vi "A33ConfigureAM.vi"(0 "VISA resource name":refnum<visa-resource-name>, 1 "Enable Amplitude Modulation (T:Enable)":bool=TRUE, 2 "Modulation Frequency (1000.0 Hz)":dbl=1000.0 format="%#_12g", 5 "Channel (1: Channel1)":u16(ring)=1 items=["Channel1"=1, "Channel2"=2], 7 "AM Source (0: Internal)":u16(ring) items=["Internal", "External", "Channel 1", "Channel 2"], 9 "Modulation Waveform (0: Sine)":u16(ring) items=["Sine", "Square", "Triangle", "Ramp", "Negative Ramp", "Noise", "PRBS", "ARB"], 11 "error in (no error)":errorcluster, 13 "Modulation Depth (100.0 %)":dbl=100.0 format="%#_12g", 14 "Enable Carrier Suppression (F: Disable)":bool) -> (4 "VISA resource name out":refnum<visa-resource-name>, 15 "error out":errorcluster)   [LabVIEW 2022 SP3]
doc: "Configures and enables amplitude modulation (AM). In AM, the amplitude of the carrier is varied by the amplitude of the modulating waveform. \n\n<B>Note:</B> The carrier waveform shape and parameters are set by the Configure Standard Waveform VI."
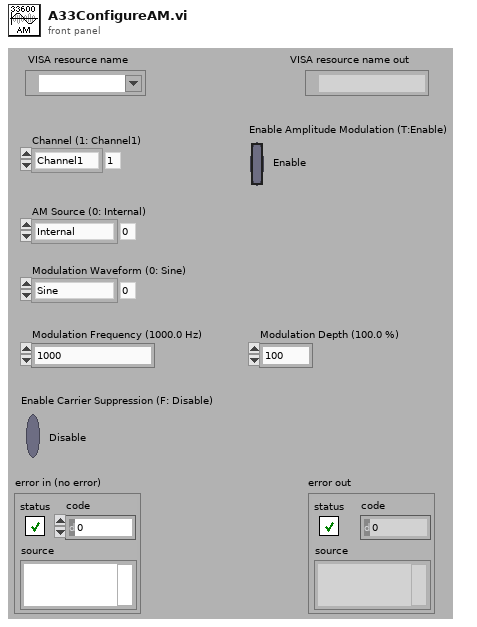
[diagram p1: front panel]
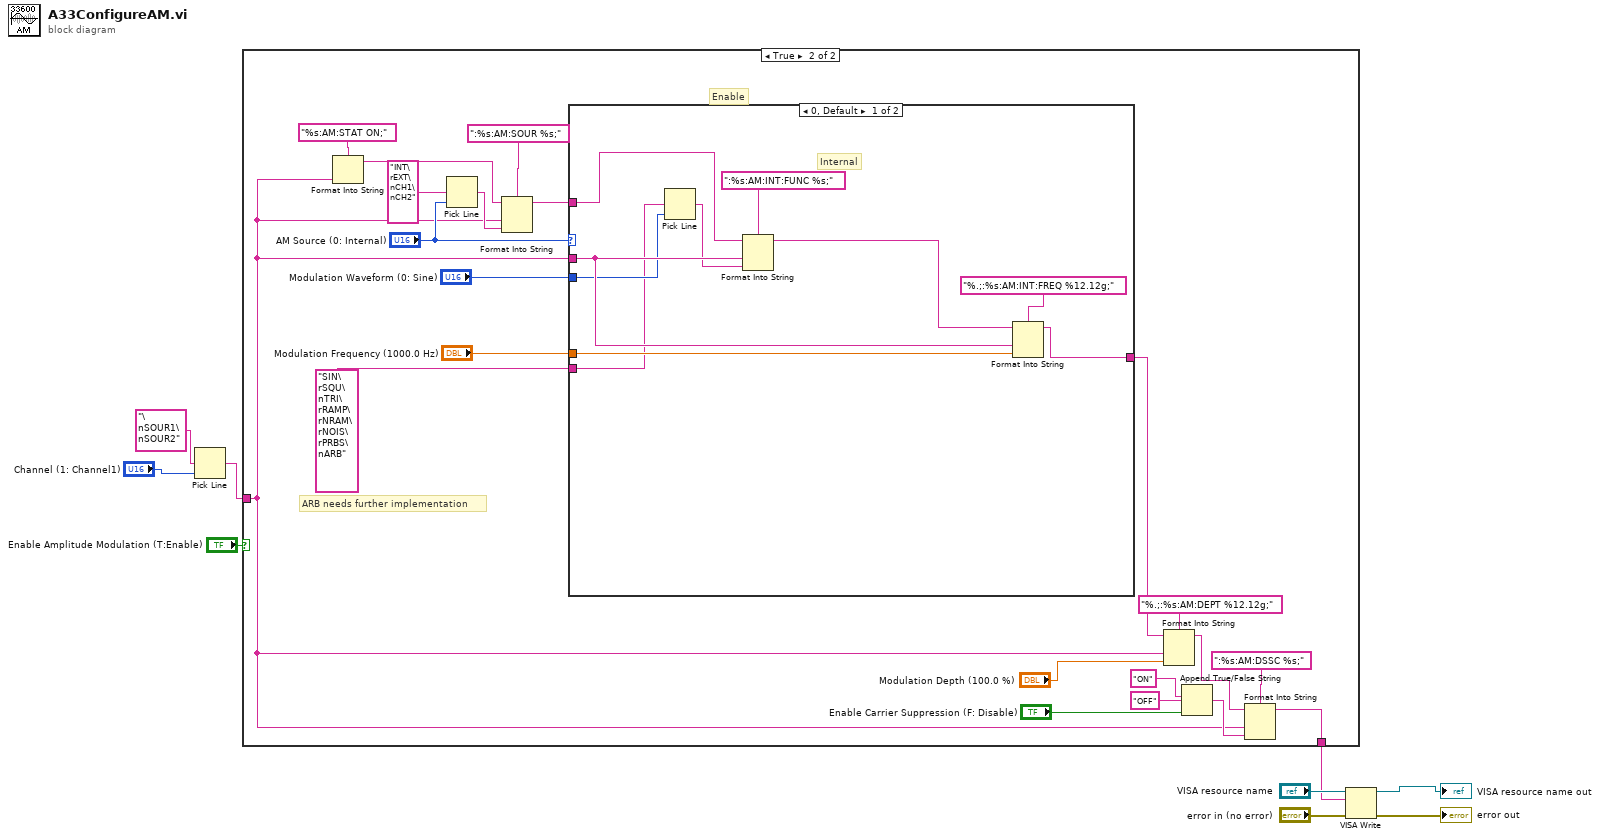
[diagram p0: block diagram]
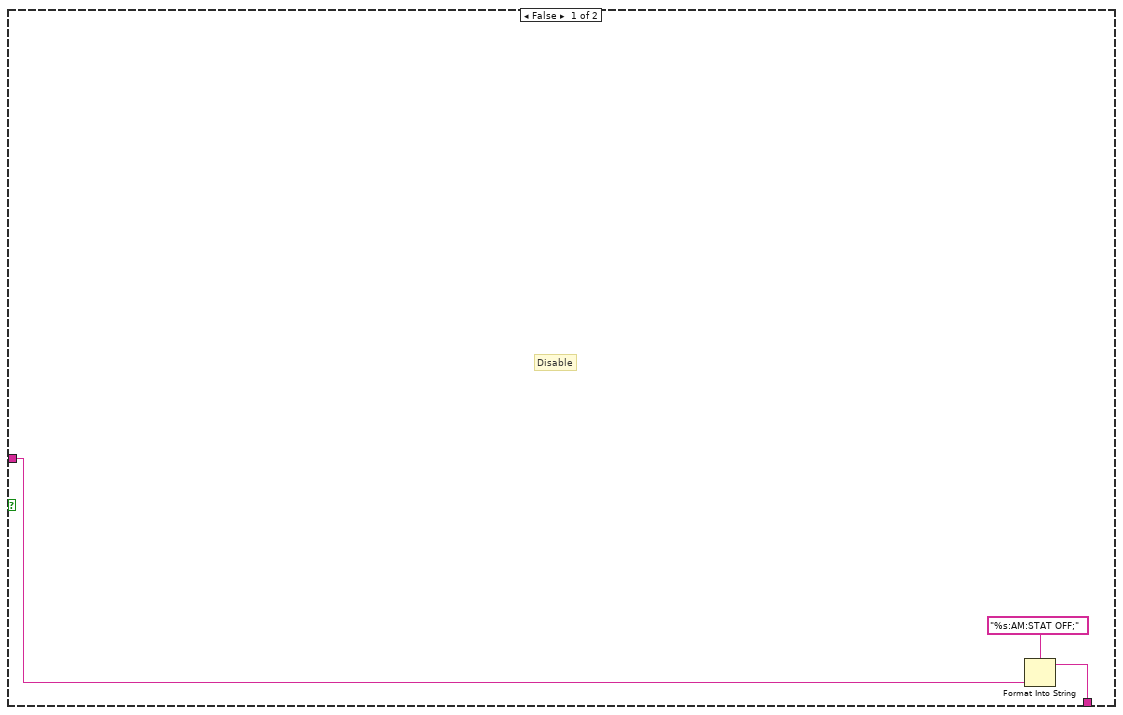
[diagram p2: hidden frame]
diagram:
  n1 = Pick Line(multi-line string="\nSOUR1\nSOUR2" ("string (\"\")"), line index="Channel (1: Channel1)") -> (output string=w1:string)  [unwired: 1 in]
  n2 = case shown="True" "Enable Amplitude Modulation (T:Enable)" {
    tunnel: [w11 w15] -> w7
    tunnel: w1 -> [w10 w13]
    frame False {
      # "Disable"
      n3 = Format Into String(format string="%s:AM:STAT OFF;", w10) -> (resulting string=w11:string)  [unwired: 2 in, 1 out]
    }
    frame True {
      # "ARB needs further implementation"
      # "Enable"
      n4 = Format Into String(format string="%s:AM:STAT ON;", w13) -> (resulting string=w16:string)  [unwired: 2 in, 1 out]
      n5 = Pick Line(multi-line string="INT\rEXT\nCH1\nCH2", line index="AM Source (0: Internal)") -> (output string=w18:string)  [unwired: 1 in]
      n6 = Format Into String(format string=":%s:AM:SOUR %s;", initial string=w16, w13, w18) -> (resulting string=w20:string)  [unwired: 1 in, 1 out]
      n7 = case shown="0, Default" "AM Source (0: Internal)" {
        tunnel: w13 -> [w39 _]
        tunnel: [w41 w44] -> w32
        tunnel: "Modulation Waveform (0: Sine)" -> [w36 _]
        tunnel: "Modulation Frequency (1000.0 Hz)" -> [w40 _]
        tunnel: w20 -> [w37 w44]
        tunnel: "SIN\rSQU\nTRI\rRAMP\rNRAM\rNOIS\rPRBS\nARB" -> [w35 _]
        frame 0, Default {
          # "Internal"
          n8 = Pick Line(multi-line string=w35, line index=w36) -> (output string=w38:string)  [unwired: 1 in]
          n9 = Format Into String(format string=":%s:AM:INT:FUNC %s;", initial string=w37, w39, w38) -> (resulting string=w34:string)  [unwired: 1 in, 1 out]
          n10 = Format Into String(format string="%.;:%s:AM:INT:FREQ %12.12g;", initial string=w34, w39, w40) -> (resulting string=w41:string)  [unwired: 1 in, 1 out]
        }
        frame 1..3 {
          # "Other Channel or External"
        }
      }
      n11 = Format Into String(format string="%.;:%s:AM:DEPT %12.12g;", initial string=w32, w13, "Modulation Depth (100.0 %)") -> (resulting string=w28:string)  [unwired: 1 in, 1 out]
      n12 = Append True/False String(1:"Enable Carrier Suppression (F: Disable)", 2:"OFF", 3:"ON") -> (0:w23:string)  [unwired: 1 in]
      n13 = Format Into String(format string=":%s:AM:DSSC %s;", initial string=w28, w13, w23) -> (resulting string=w15:string)  [unwired: 1 in, 1 out]
    }
  }
  n14 = VISA Write(VISA resource name="VISA resource name", write buffer=w7, error in (no error)="error in (no error)") -> (VISA resource name out=→"VISA resource name out":refnum<visa-resource-name>, error out=→"error out":errorcluster)  [unwired: 1 out]
